vi "Read Show UI.vi"(8 "error in (no error)":errorcluster, 11 "UI Data in":refnum<class "Settings UI.lvclass">) -> (0 "error out":errorcluster, 2 "Show UI":bool, 3 "UI Data out":refnum<class "Settings UI.lvclass">)   [LabVIEW 2020, in "Output Sequencer.lvlib" / "Settings UI.lvclass"]
uses:
  Settings UI.lvclass
  Settings UI.lvclass/Settings UI.ctl
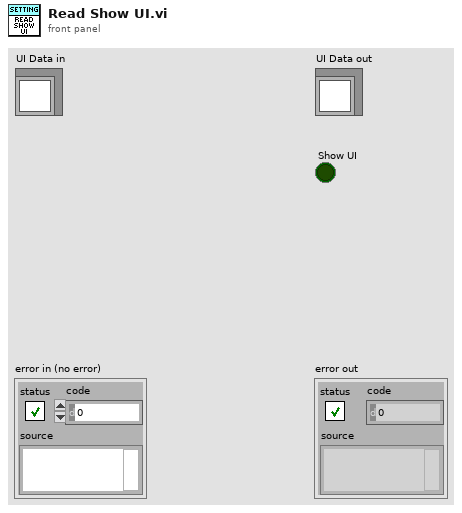
[diagram p1: front panel]
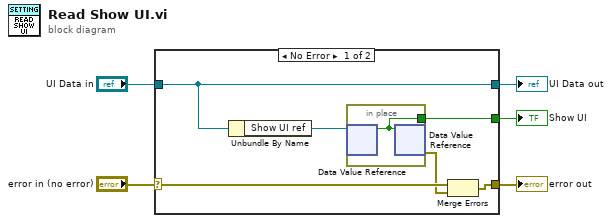
[diagram p0: block diagram]
diagram:
  n1 = case shown="No Error" "error in (no error)" {
    selector: "error in (no error)" -> [w8 w13]
    tunnel: [w6 w13] -> w4
    tunnel: [w11 w14] -> w2
    tunnel: "UI Data in" -> [w11 w14]
    tunnel: [w9 _] -> w1
    frame No Error {
      n2 = Unbundle By Name(w11) -> ("Show UI ref"=w10:refnum<data-value>)
      n3 = in-place {
        in-place-border: [w12] -> w9
        n4 = in-place-dvr #1(w10) -> (w12:bool)  [unwired: 1 out]
        n5 = in-place-dvr #1(w12) -> (w7:errorcluster)  [unwired: 1 out]
      }
      n6 = Merge Errors(w8, w7) -> (w6:errorcluster)
    }
    frame Error {
    }
  }
  "error out" <- w4
  "UI Data out" <- w2
  "Show UI" <- w1
